vi "CreateButtonBarFlow.vi"() -> ()   [LabVIEW 2021, in "ButtonBarFlow.lvlib"]
uses:
  ButtonBarFlow.lvlib
  ActiveObjects/VerticalButtonBar/ButtonCollection/ButtonCollection.lvclass
panel:
  in  "Orientation":enum16{"Horizonal", "Vertical"}(ring)
  in  "Simplified":bool
  in  "TargetFolder":path
  out "PlantUMLText":string
  in  "Path":path
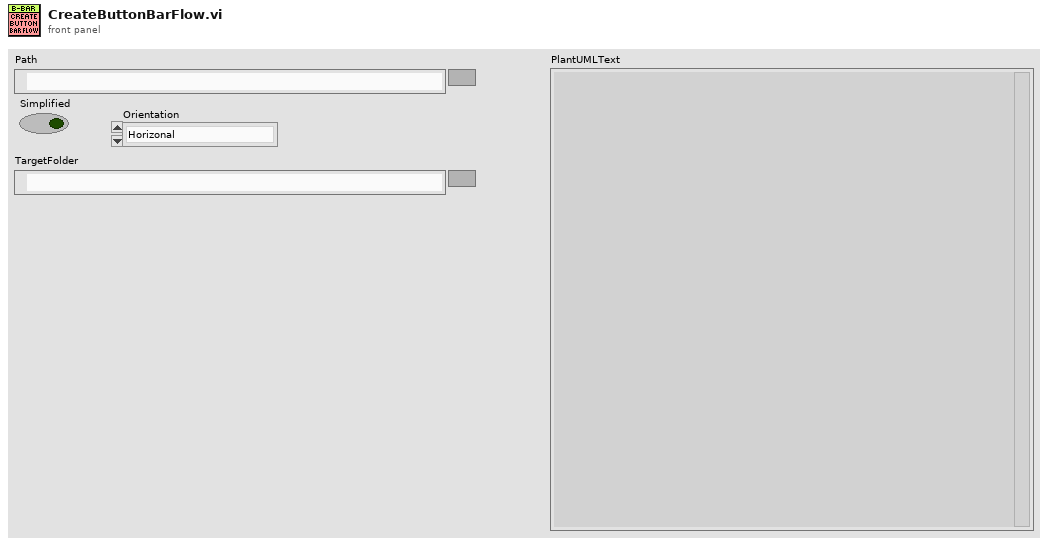
[diagram p1: front panel]
types:
  T1 = typedef "ButtonCollection.lvclass/ButtonDefinition.ctl" = cluster{"ThisNavigationName":string, "ButtonLabel":string, "Caption":string, "Tooltip":string, "EnabledExpression":string, "Actions":cluster{"ActionType":string, "TargetObject":string, "Parameter":string, "WaitUntilDone":bool}[], "NextNavigationName":string}
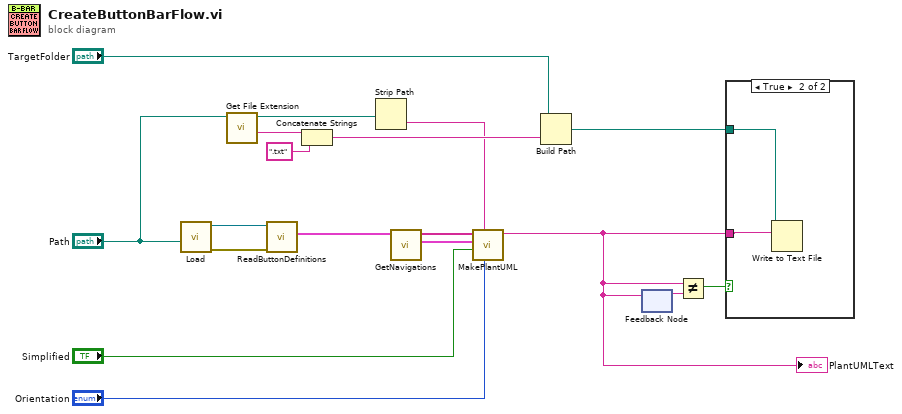
[diagram p0: block diagram]
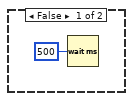
[diagram p2: hidden frame]
diagram:
  n1 = call "Load.vi"("Path"="Path") -> ("ErrorOut"=w17:errorcluster, "ObjectOut"=w16:refnum<class "ButtonCollection.lvclass">)  [unwired: 9 in]
  n2 = call <vilib>:"Get File Extension.vi"("file"="Path") -> ("filename without extension"=w14:string)  [unwired: 6 in, 4 out]
  n3 = call-dynamic "ReadButtonDefinitions.vi"("Error In"=w17, "object in"=w16) -> ("ButtonDefinitions"=w15:T1[])  [unwired: 7 in, 2 out]
  n4 = Concatenate Strings(w14, ".txt" ("string")) -> (w12:string)
  n5 = Strip Path(path="Path") -> (name=w5:string)  [unwired: 1 out]
  n6 = call "GetNavigations.vi"("ButtonDefinitions"=w15) -> ("Array"=w8:cluster{T1[]}[], "Navigations"=w7:string[])  [unwired: 9 in]
  n7 = call "MakePlantUML.vi"("Orientation"="Orientation", "DiagramName"=w5, "Simplified"="Simplified", "NavigationsDetails"=w8, "NavigationNames"=w7) -> ("PlantUMLText"=w3:string)  [unwired: 6 in]
  "PlantUMLText" <- w3
  n8 = Build Path(base path="TargetFolder", name or relative path=w12) -> (appended path=w11:path)
  n9 = feedback-in #1(w3) -> ()
  n10 = feedback #1() -> (w10:string)  [unwired: 1 in]
  n11 = Not Equal?(x=w3, y=w10) -> (x != y?=w9:bool)
  n12 = case shown="True" w9 {
    tunnel: w11 -> [_ w20]
    tunnel: w3 -> [_ w19]
    frame False {
      n13 = Wait (ms)(milliseconds to wait=u32 500) -> ()  [unwired: 1 out]
    }
    frame True {
      n14 = Write to Text File(file (use dialog)=w20, text=w19) -> ()  [unwired: 2 in, 3 out]
    }
  }
